vi "NIconTrig.vi"(3 "error in":errorcluster, 4 "Trigger":T1 {"Slope" items=["Positive", "Negative"]; "Level" format="%.2f"; "Coupling" items=["DC 1 MOhm", "AC 1 MOhm", "HF Reject", "LF Reject", "AC Plus HF Reject"]; "Source" items=["Chan 1", "External"]}, 5 "InstrumentID":refnum<k15>) -> (0 "error out":errorcluster, 2 "dup id":refnum<k15>)   [LabVIEW 2022 SP3]
uses:
  <instrlib>/niScope/Controls/niScope trigger source.ctl
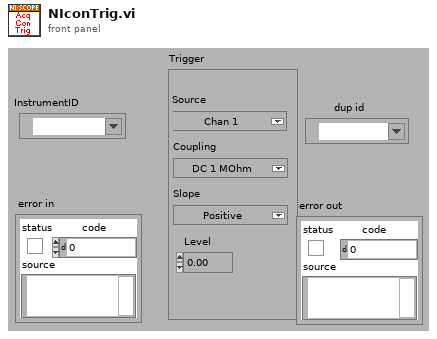
[diagram p1: front panel]
types:
  T1 = cluster{"Source":u16, "Coupling":u16, "Slope":u16, "Level":dbl}
  T2 = typedef "niScope trigger source.ctl" = string
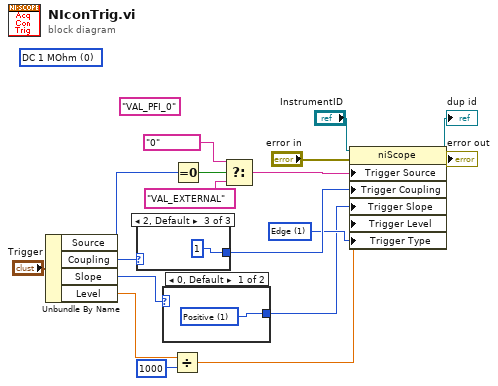
[diagram p0: block diagram]
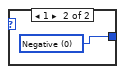
[diagram p2: hidden frame]
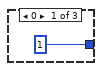
[diagram p3: hidden frame]
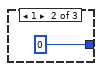
[diagram p4: hidden frame]
diagram:
  (unwired) u16 0 items=["DC 1 MOhm", "AC 1 MOhm", "DC 50 Ohm", "AC 50 Ohm"] ("Coupling")
  (unwired) "VAL_PFI_0"
  w4 = 1 items=["Edge"=1, "Video"=5, "Immediate"=6, "Hysteresis"=1001, "Digital"=1002, "Window"=1003, "Software"=1004] ("Triggering:Trigger Type")
  n1 = Unbundle By Name("Trigger") -> ("Source"=w18:u16, "Coupling"=w13:u16, "Slope"=w3:u16, "Level"=w12:dbl)
  n2 = case shown="2, Default" w13 {
    tunnel: [1 0 1] -> w9
    frame 0 {
    }
    frame 1 {
    }
    frame 2, Default {
    }
  }
  n3 = case shown="0, Default" w3 {
    tunnel: [w22 w23] -> w2
    frame 0, Default {
      w22 = 1 items=["Positive"=1, "Negative"=0] ("Triggering:Trigger Slope")
    }
    frame 1 {
      w23 = 0 items=["Positive"=1, "Negative"=0] ("Triggering:Trigger Slope")
    }
  }
  n4 = Divide(x=w12, y=1000) -> (x/y=w8:dbl)
  n5 = Equal To 0?(x=w18) -> (x = 0?=w16:bool)
  n6 = Select(t=T2 "0" ("trigger source"), s=w16, f=T2 "VAL_EXTERNAL" ("trigger source")) -> (s? t:f=w1:T2)
  n7 = property class="niScope"(reference="InstrumentID", error in="error in", "Trigger Source"=w1, "Trigger Coupling"=w9, "Trigger Slope"=w2, "Trigger Level"=w8, "Trigger Type"=w4) -> (reference out=→"dup id":refnum<k15>, error out=→"error out":errorcluster)
